vi "ExtractXML.vi"() -> ()   [LabVIEW 2014]
uses:
  ZLIB/lvzip.llb/ZLIB Open Unzip Archive__ogtk.vi
  ZLIB/lvzip.llb/ZLIB Extract Stream__ogtk.vi
  ZLIB/ZLIB.lvlib
panel:
  out "byte stream":string="<?xml version=\"1.0\" encoding=\"UTF-8\"?>\n<office:document-content xmlns:office=\"urn:oasis:names:tc:opendocument:xmlns:office:1.0\" xmlns:style=\"urn:oasis:names:tc:opendocument:xmlns:style:1.0\" xmlns:text=\"urn:oasis:names:tc:opendocument:xmlns:text:1.0\" xmlns:table=\"urn:oasis:names:tc:opendocument:xmlns:table:1.0\" xmlns:draw=\"urn:oasis:names:tc:opendocument:xmlns:drawing:1.0\" xmlns:fo=\"urn:oasis:names:tc:opendocument:xmlns:xsl-fo-compatible:1.0\" xmlns:xlink=\"http://www.w3.org/1999/xlink\" xmlns:dc=\"http://purl.org/dc/elements/1.1/\" xmlns:meta=\"urn:oasis:names:tc:opendocument:xmlns:meta:1.0\" xmlns:number=\"urn:oasis:names:tc:opendocument:xmlns:datastyle:1.0\" xmlns:presentation=\"urn:oasis:names:tc:opendocument:xmlns:presentation:1.0\" xmlns:svg=\"urn:oasis:names:tc:opendocument:xmlns:svg-compatible:1.0\" xmlns:chart=\"urn:oasis:names:tc:opendocument:xmlns:chart:1.0\" xmlns:dr3d=\"urn:oasis:names:tc:opendocument:xmlns:dr3d:1.0\" xmlns:math=\"http://www.w3.org/1998/Math/MathML\" xmlns:form=\"urn:oasis:names:tc:opendocument:xmlns:form:1.0\" xmlns:script=\"urn:oasis:names:tc:opendocument:xmlns:script:1.0\" xmlns:ooo=\"http://openoffice.org/2004/office\" xmlns:ooow=\"http://openoffice.org/2004/writer\" xmlns:oooc=\"http://openoffice.org/2004/calc\" xmlns:dom=\"http://www.w3.org/2001/xml-events\" xmlns:xforms=\"http://www.w3.org/2002/xforms\" xmlns:xsd=\"http://www.w3.org/2001/XMLSchema\" xmlns:xsi=\"http://www.w3.org/2001/XMLSchema-instance\" xmlns:rpt=\"http://openoffice.org/2005/report\" xmlns:of=\"urn:oasis:names:tc:opendocument:xmlns:of:1.2\" xmlns:xhtml=\"http://www.w3.org/1999/xhtml\" xmlns:grddl=\"http://www.w3.org/2003/g/data-view#\" xmlns:tableooo=\"http://openoffice.org/2009/table\" xmlns:drawooo=\"http://openoffice.org/2010/draw\" xmlns:calcext=\"urn:org:documentfoundation:names:experimental:calc:xmlns:calcext:1.0\" xmlns:loext=\"urn:org:documentfoundation:names:experimental:office:xmlns:loext:1.0\" xmlns:field=\"urn:openoffice:names:experimental:ooo-ms-interop:xmlns:field:1.0\" xmlns:formx=\"urn:openoffice:names:experimental:ooxml-odf-interop:xmlns:form:1.0\" xmlns:css3t=\"http://www.w3.org/TR/css3-text/\" office:version=\"1.2\"><office:scripts/><office:font-face-decls><style:font-face style:name=\"Arial\" svg:font-family=\"Arial\" style:font-family-generic=\"swiss\" style:font-pitch=\"variable\"/><style:font-face style:name=\"Mangal\" svg:font-family=\"Mangal\" style:font-family-generic=\"system\" style:font-pitch=\"variable\"/><style:font-face style:name=\"Microsoft YaHei\" svg:font-family=\"&apos;Microsoft YaHei&apos;\" style:font-family-generic=\"system\" style:font-pitch=\"variable\"/><style:font-face style:name=\"Segoe UI\" svg:font-family=\"&apos;Segoe UI&apos;\" style:font-family-generic=\"system\" style:font-pitch=\"variable\"/><style:font-face style:name=\"Tahoma\" svg:font-family=\"Tahoma\" style:font-family-generic=\"system\" style:font-pitch=\"variable\"/></office:font-face-decls><office:automatic-styles><style:style style:name=\"co1\" style:family=\"table-column\"><style:table-column-properties fo:break-before=\"auto\" style:column-width=\"2.258cm\"/></style:style><style:style style:name=\"co2\" style:family=\"table-column\"><style:table-column-properties fo:break-before=\"auto\" style:column-width=\"5.999cm\"/></style:style><style:style style:name=\"ro1\" style:family=\"table-row\"><style:table-row-properties style:row-height=\"0.453cm\" fo:break-before=\"auto\" style:use-optimal-row-height=\"true\"/></style:style><style:style style:name=\"ro2\" style:family=\"table-row\"><style:table-row-properties style:row-height=\"0.473cm\" fo:break-before=\"auto\" style:use-optimal-row-height=\"true\"/></style:style><style:style style:name=\"ta1\" style:family=\"table\" style:master-page-name=\"Default\"><style:table-properties table:display=\"true\" style:writing-mode=\"lr-tb\"/></style:style></office:automatic-styles><office:body><office:spreadsheet><table:table table:name=\"Sheet1\" table:style-name=\"ta1\"><table:table-column table:style-name=\"co1\" table:default-cell-style-name=\"Default\"/><table:table-column table:style-name=\"co2\" table:default-cell-style-name=\"Default\"/><table:table-column table:style-name=\"co1\" table:number-columns-repeated=\"11\" table:default-cell-style-name=\"Default\"/><table:table-row table:style-name=\"ro1\"><table:table-cell office:value-type=\"string\" calcext:value-type=\"string\"><text:p>Title1</text:p></table:table-cell><table:table-cell table:number-columns-repeated=\"12\"/></table:table-row><table:table-row table:style-name=\"ro2\"><table:table-cell/><table:table-cell office:value-type=\"string\" calcext:value-type=\"string\"><text:p>aaaaaaaaaaaaaaaaaaaaa</text:p></table:table-cell><table:table-cell table:number-columns-repeated=\"5\"/><table:table-cell office:value-type=\"string\" calcext:value-type=\"string\"><text:p>H2</text:p></table:table-cell><table:table-cell table:number-columns-repeated=\"5\"/></table:table-row><table:table-row table:style-name=\"ro2\"><table:table-cell/><table:table-cell office:value-type=\"string\" calcext:value-type=\"string\"><text:p>bbbbbbbbbbbbbbbbbbbbb</text:p></table:table-cell><table:table-cell table:number-columns-repeated=\"11\"/></table:table-row><table:table-row table:style-name=\"ro2\"><table:table-cell/><table:table-cell office:value-type=\"string\" calcext:value-type=\"string\"><text:p>ccccccccccccccccccccc</text:p></table:table-cell><table:table-cell table:number-columns-repeated=\"11\"/></table:table-row><table:table-row table:style-name=\"ro2\"><table:table-cell/><table:table-cell office:value-type=\"string\" calcext:value-type=\"string\"><text:p>ddddddddddddddddddddd</text:p></table:table-cell><table:table-cell table:number-columns-repeated=\"11\"/></table:table-row><table:table-row table:style-name=\"ro1\"><table:table-cell office:value-type=\"string\" calcext:value-type=\"string\"><text:p>Title2</text:p></table:table-cell><table:table-cell table:number-columns-repeated=\"12\"/></table:table-row><table:table-row table:style-name=\"ro2\"><table:table-cell/><table:table-cell office:value-type=\"string\" calcext:value-type=\"string\"><text:p>eeeeeeeeeeeeeeeeeeeee</text:p></table:table-cell><table:table-cell table:number-columns-repeated=\"11\"/></table:table-row><table:table-row table:style-name=\"ro2\"><table:table-cell/><table:table-cell office:value-type=\"string\" calcext:value-type=\"string\"><text:p>ffffffffffffffffffffffffffffffffffffffff</text:p></table:table-cell><table:table-cell table:number-columns-repeated=\"11\"/></table:table-row><table:table-row table:style-name=\"ro1\"><table:table-cell/><table:table-cell office:value-type=\"string\" calcext:value-type=\"string\"><text:p>ggggggggggggggggggggg</text:p></table:table-cell><table:table-cell table:number-columns-repeated=\"11\"/></table:table-row><table:table-row table:style-name=\"ro1\" table:number-rows-repeated=\"5\"><table:table-cell table:number-columns-repeated=\"13\"/></table:table-row><table:table-row table:style-name=\"ro1\"><table:table-cell table:number-columns-repeated=\"4\"/><table:table-cell office:value-type=\"string\" calcext:value-type=\"string\"><text:p>E16</text:p></table:table-cell><table:table-cell table:number-columns-repeated=\"8\"/></table:table-row><table:table-row table:style-name=\"ro1\" table:number-rows-repeated=\"10\"><table:table-cell table:number-columns-repeated=\"13\"/></table:table-row><table:table-row table:style-name=\"ro1\"><table:table-cell table:number-columns-repeated=\"12\"/><table:table-cell office:value-type=\"string\" calcext:value-type=\"string\"><text:p>M26</text:p></table:table-cell></table:table-row></table:table><table:named-expressions/></office:spreadsheet></office:body></office:document-content>"
  in  "archive name":path=path "C:/Users/Steve Watts/Desktop/ISO9000/Checklist/eee - Copy.ods"
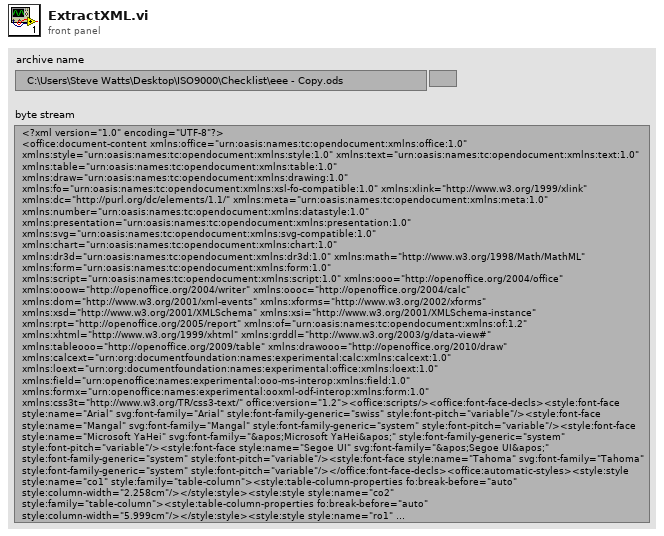
[diagram p1: front panel]
types:
  T1 = typedef "ZLIB.lvlib/ZLIB Unzip Handle__ogtk.ctl" = refnum<k1>
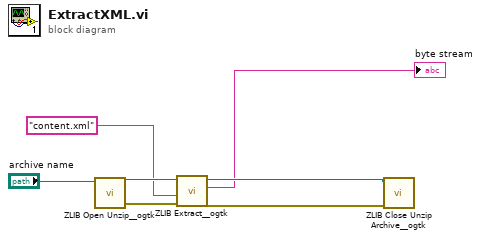
[diagram p0: block diagram]
diagram:
  n1 = call-poly "ZLIB Open Unzip__ogtk.vi"("archive name"="archive name") -> ("error out"=w6:errorcluster, "unzip Refnum"=w5:T1)  [unwired: 5 in]
  n2 = call-poly "ZLIB Extract__ogtk.vi"("error in (no error)"=w6, "internal name"="content.xml" ("name (empty: -)"), "unzip Refnum"=w5) -> ("error out"=w2:errorcluster, "byte stream"=→"byte stream":string, "unzip Refnum out"=w3:T1)  [unwired: 4 in]
  n3 = call "ZLIB Close Unzip Archive__ogtk.vi"("error in (no error)"=w2, "unzip Refnum"=w3) -> ()  [unwired: 5 in, 1 out]
